vi "Trim Whitespace (String) 1.vi"(5 "Remove non-printable characters":bool, 7 "Remove (leading and trailing)":enum16{"leading", "trailing", "both"}(ring)=enum."both", 8 "String in":string) -> (2 "String out":string)   [LabVIEW 2009]
doc: "Removes leading and/or trailing whitespace from a string.\nWhitespace is defined as any of the following characters \\s \\t \\n \\0B \\f \\r.\nNon-printable is defined as any character less than ASCII 0x21.\n\nThis VI 's execution is set to <b>subroutine</b>\nThis VI is <b>reentrant</b>"
panel:
  # "Trim Whitespace (String) 1.vi\n\nRemoves leading and/or trailing whitespace from a string.\n\nPlease visit http://www.OpenG.org to learn about the\nOpen Source LabVIEW software movement.\n\nNOTICE -- YOU MUST LEAVE THIS NOTICE IN PLACE.  PER THE TERMS OF THE LICENSE BELOW, YOU MAY SUBLICENSE THIS SOFTWARE \nIN ANY WAY THAT DOES NOT CONFLICT WITH THIS LICENSE.\n\n### BSD License (http://www.opensource.org/licenses/bsd-license.php) Begin ###\n\nCopyright (c) 2002-2006, Jim Kring <jim@jimkring.com>\nCopyright (c) 2002, Cal-Bay Systems, Inc. <info@calbay.com>\nCopyright (c) 2011 -  Shaun Rumbell <shaunr@labview-tools.com> \nCopyright (c) 2011 - Jonathon Green <jg@jgcode.net>\n\nAll rights reserved.\n\nRedistribution and use in source and binary forms, with or without modification, are permitted provided that the following conditions are met:\n\n    * Redistributions of source code must retain the above copyright notice, this list of conditions and the following disclaimer.\n    * Redistributions in binary form must reproduce the above copyright notice, this list of conditions and the following disclaimer in the \n       documentation and/or other materials provided with the distribution.\n    * Neither the name of SciWare, James Kring, Inc., nor the names of its contributors may be used to endorse or promote products derived \n       from this software without specific prior written permission.\n\nTHIS SOFTWARE IS PROVIDED BY THE COPYRIGHT HOLDERS AND CONTRIBUTORS \"AS IS\" AND ANY EXPRESS OR IMPLIED WARRANTIES, \nINCLUDING, BUT NOT LIMITED TO, THE IMPLIED WARRANTIES OF MERCHANTABILITY AND FITNESS FOR A PARTICULAR PURPOSE ARE \nDISCLAIMED. IN NO EVENT SHALL THE COPYRIGHT OWNER OR CONTRIBUTORS BE LIABLE FOR ANY DIRECT, INDIRECT, INCIDENTAL,\n SPECIAL, EXEMPLARY, OR CONSEQUENTIAL DAMAGES (INCLUDING, BUT NOT LIMITED TO, PROCUREMENT OF SUBSTITUTE GOODS OR \nSERVICES; LOSS OF USE, DATA, OR PROFITS; OR BUSINESS INTERRUPTION) HOWEVER CAUSED AND ON ANY THEORY OF LIABILITY, \nWHETHER IN CONTRACT, STRICT LIABILITY, OR TORT (INCLUDING NEGLIGENCE OR OTHERWISE) ARISING IN ANY WAY OUT OF THE USE \nOF THIS SOFTWARE, EVEN IF ADVISED OF THE POSSIBILITY OF SUCH DAMAGE.\n\n### BSD License End ###"
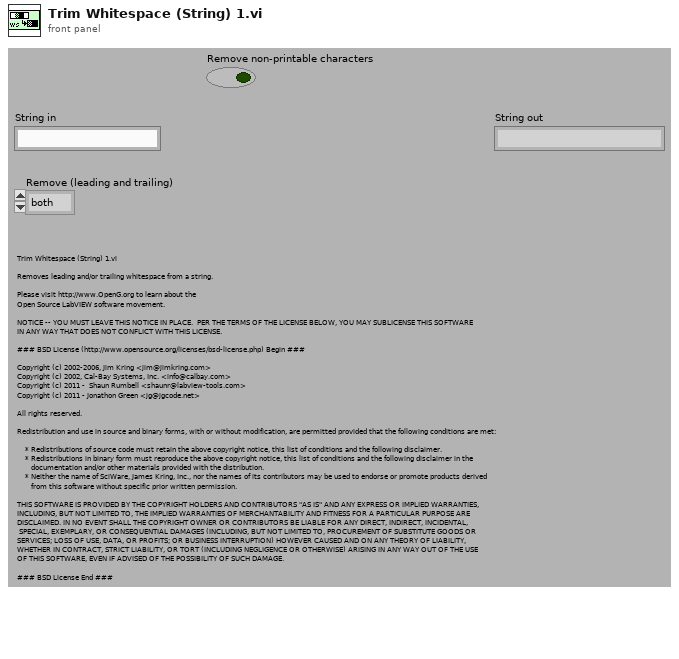
[diagram p1: front panel]
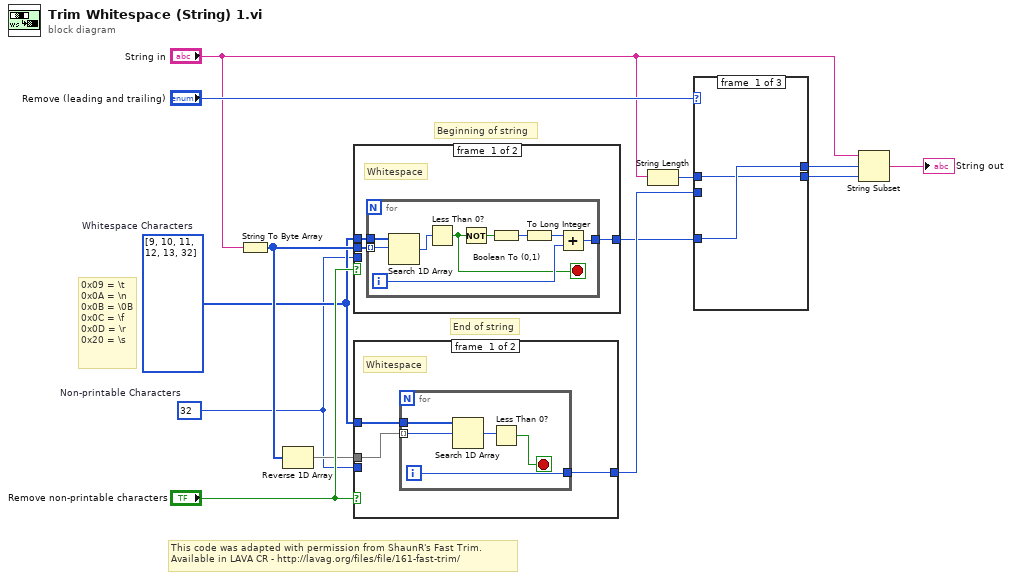
[diagram p0: block diagram]
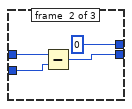
[diagram p2: hidden frame]
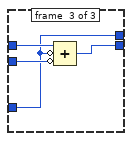
[diagram p3: hidden frame]
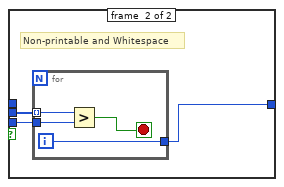
[diagram p4: hidden frame]
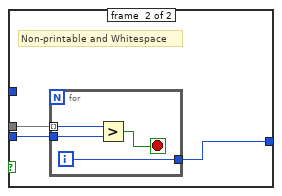
[diagram p5: hidden frame]
diagram:
  w1 = u8 32  # Non-printable Characters
  w2 = u8[] [9, 10, 11, 12, 13, 32]  # Whitespace Characters
  # "This code was adapted with permission from ShaunR's Fast Trim. \nAvailable in LAVA CR - http://lavag.org/files/file/161-fast-trim/"
  # "0x09 = \\t\n0x0A = \\n\n0x0B = \\0B\n0x0C = \\f\n0x0D = \\r\n0x20 = \\s"
  # "Beginning of string"
  # "End of string"
  n1 = String To Byte Array(string="String in") -> (unsigned byte array=w9:u8[])
  n2 = Reverse 1D Array(array=w9) -> (reversed array=w10:u8[])
  n3 = case shown="False" "Remove non-printable characters" {
    tunnel: w9 -> [w16 w28]
    tunnel: [w15 w27] -> w4
    tunnel: w2 -> [w14 _]
    tunnel: w1 -> [_ w26]
    frame #0 {
      # "Whitespace"
      n4 = for {
        tunnel: w16 -> [w24] mode=indexing
        tunnel: [w21] -> w15
        tunnel: w14 -> [w17]
        i -> [w25]
        stop <- w22 stop-if-true
        n5 = Search 1D Array(1D array=w17, element=w24) -> (index of element=w23:i32)  [unwired: 1 in]
        n6 = Less Than 0?(x=w23) -> (x < 0?=w22:bool)
        n7 = Not(x=w22) -> (.not. x?=w19:bool)
        n8 = Boolean To (0,1)(Boolean=w19) -> (0, 1=w20:i16)
        n9 = To Long Integer(number=w20) -> (32bit integer=w18:i32)
        n10 = Add(x=w18, y=w25) -> (x+y=w21:i32)
      }
    }
    frame #1 {
      # "Non-printable and Whitespace"
      n11 = for {
        tunnel: w28 -> [w32] mode=indexing
        tunnel: [w30] -> w27
        tunnel: w26 -> [w29]
        i -> [w30]
        stop <- w31 stop-if-true
        n12 = Greater?(x=w32, y=w29) -> (0:w31:bool)
      }
    }
  }
  n13 = case shown="True" "Remove non-printable characters" {
    tunnel: w10 -> [w35 w43]
    tunnel: [w34 w42] -> w5
    tunnel: w2 -> [w33 _]
    tunnel: w1 -> [_ w41]
    frame #0 {
      # "Whitespace"
      n14 = for {
        tunnel: w35 -> [w39] mode=indexing
        tunnel: [w40] -> w34
        tunnel: w33 -> [w36]
        i -> [w40]
        stop <- w37 stop-if-true
        n15 = Search 1D Array(1D array=w36, element=w39) -> (index of element=w38:i32)  [unwired: 1 in]
        n16 = Less Than 0?(x=w38) -> (x < 0?=w37:bool)
      }
    }
    frame #1 {
      # "Non-printable and Whitespace"
      n17 = for {
        tunnel: w43 -> [w47] mode=indexing
        tunnel: [w45] -> w42
        tunnel: w41 -> [w44]
        i -> [w45]
        stop <- w46 stop-if-true
        n18 = Greater?(x=w47, y=w44) -> (0:w46:bool)
      }
    }
  }
  n19 = String Length(string="String in") -> (length=w6:i32)
  n20 = case shown="\"both\"" "Remove (leading and trailing)" {
    tunnel: [w48 w50 w55] -> w8
    tunnel: [w49 0 w54] -> w7
    tunnel: w4 -> [w49 _ w54]
    tunnel: w6 -> [w48 w52 w57]
    tunnel: w5 -> [_ w51 w56]
    frame #0 {
    }
    frame #1 {
      n21 = Subtract(x=w52, y=w51) -> (x-y=w50:i32)
    }
    frame #2 {
      n22 = Compound Arithmetic op=ADD(w57, invert w54, invert w56) -> (w55:i32)
    }
  }
  n23 = String Subset(string="String in", offset (0)=w7, length (rest)=w8) -> (substring=→"String out":string)
